vi "Configure - Digital.vi"(5 "master clock channel list":string, 7 "data channel list":string, 8 "error in (no error)":errorcluster, 9 "signal settings":T9, 10 "digital protocol settings":T1={"logic level"=enum."3.3 V", "PCM Data Configuration"={"Frame Sync Edge for Channel 0"=enum."Falling", "Channel Count Per Frame"=2, "Channel Length"=32, "Bit Depth"=24, "Channel 0 Offset"=1, "Endianness"=enum."MSB First", "Data Justification"=enum."Left Justified"}, "bit clock rate"=3025000.0, "master clock rate"=3025000.0, "clock mode"=enum."divided clock", "Frame Sync Clock Control"={"Frame Length"=64, "Frame Sync Pulse Width"=32, "Bit Clock Edge  Sync"=enum."Falling"}} {"master clock rate" format="%.4p"; "bit clock rate" format="%.4p"}, 11 "AudioGeneration in":refnum<class "AudioGeneration.lvclass">) -> (0 "error out":errorcluster, 3 "AudioGeneration out":refnum<class "AudioGeneration.lvclass">)   [LabVIEW 2021, in "AudioGeneration.lvclass"]
uses:
  AudioGeneration.lvclass
  AudioGeneration.lvclass/AudioGeneration.ctl
  <vilib>/NI/STM/TCP/TCP Write Options.ctl
  <vilib>/NI/STM/NI STM.lvlib
  controls/generation type.ctl
  controls/AudioGenTypeDefs.lvlib
  <vilib>/PDM Acquisition Toolkit/host/Classes/Session/Controls/Logic Levels.ctl
  <vilib>/PDM Acquisition Toolkit/host/Classes/Session/DecoderSession.lvclass
  <vilib>/PDM Acquisition Toolkit/shared/controls/Digital Edge.ctl
  <vilib>/PDM Acquisition Toolkit/shared/PDM Shared.lvlib
  <vilib>/PDM Acquisition Toolkit/shared/controls/PCM Bit Endianness.ctl
  <vilib>/PDM Acquisition Toolkit/shared/controls/PCM Data Justification.ctl
  <vilib>/PDM Acquisition Toolkit/shared/controls/PCM Data Format Configuration.ctl
  <vilib>/PDM Acquisition Toolkit/shared/controls/clock mode.ctl
  <vilib>/PDM Acquisition Toolkit/shared/controls/PCM Frame Sync Control.ctl
  controls/digital protocol settings.ctl
  controls/signal type.ctl
  controls/signal settings.ctl
  controls/digital generation settings.ctl
  <vilib>/NI/STM/TCP/Write Message (TCP).vi
  shared/controls/digital output level units.ctl
  shared/controls/audio controls.lvlib
panel:
  out "timeout":bool
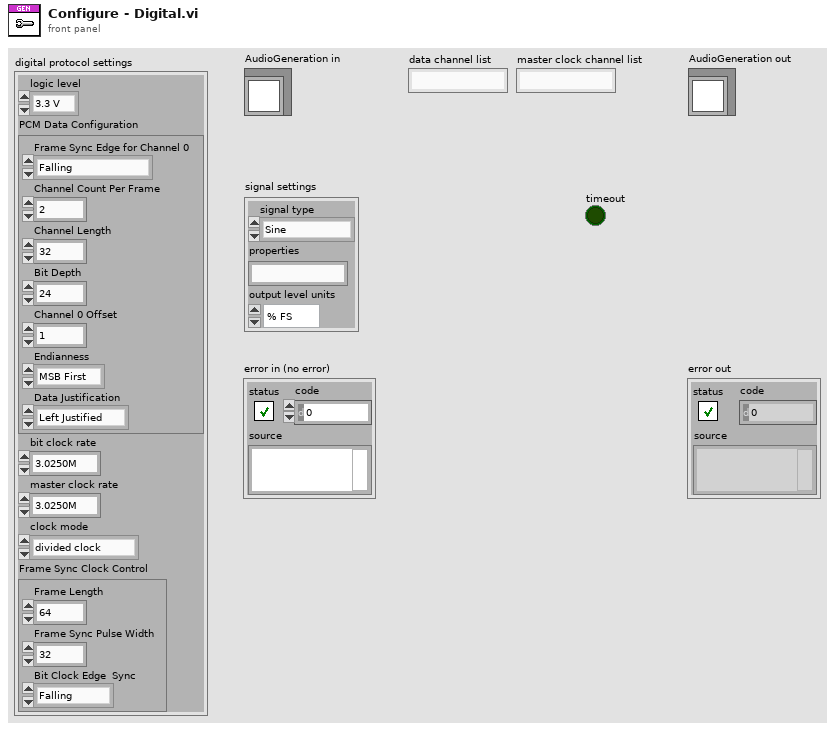
[diagram p1: front panel]
types:
  T1 = typedef "AudioGenTypeDefs.lvlib/digital protocol settings.ctl" = cluster{"logic level":T2, "PCM Data Configuration":T3, "bit clock rate":sgl, "master clock rate":sgl, "clock mode":T7, "Frame Sync Clock Control":T8}
  T2 = typedef "PDM Acquisition Class Library.lvlib/DecoderSession.lvclass/Logic Levels.ctl" = enum16{"3.3 V", "1.8 V", "1.2 V"}
  T3 = typedef "PDM Shared.lvlib/PCM Data Format Configuration.ctl" = cluster{"Frame Sync Edge for Channel 0":T4, "Channel Count Per Frame":u8, "Channel Length":u16, "Bit Depth":u8, "Channel 0 Offset":u16, "Endianness":T5, "Data Justification":T6}
  T4 = typedef "PDM Shared.lvlib/Digital Edge.ctl" = enum8{"Rising", "Falling"}
  T5 = typedef "PDM Shared.lvlib/PCM Bit Endianness.ctl" = enum16{"MSB First", "LSB First"}
  T6 = typedef "PDM Shared.lvlib/PCM Data Justification.ctl" = enum16{"Left Justified", "Right Justified"}
  T7 = typedef "PDM Shared.lvlib/clock mode.ctl" = enum16{"divided clock", "DDS"}
  T8 = typedef "PDM Shared.lvlib/PCM Frame Sync Control.ctl" = cluster{"Frame Length":u16, "Frame Sync Pulse Width":u16, "Bit Clock Edge  Sync":T4}
  T9 = typedef "AudioGenTypeDefs.lvlib/signal settings.ctl" = cluster{"signal type":T10, "properties":string, "output level units":T11}
  T10 = typedef "AudioGenTypeDefs.lvlib/signal type.ctl" = enum16{"Sine", "Dual Tone"}
  T11 = typedef "audio controls.lvlib/digital output level units.ctl" = enum32{"% FS", "dBFS", "V"}
  T12 = typedef "AudioGenTypeDefs.lvlib/digital generation settings.ctl" = cluster{"data channel list":string, "master clock channel list":string, "digital protocol settings":T1, "signal settings":T9}
  T13 = typedef "AudioGenTypeDefs.lvlib/generation type.ctl" = enum16{"analog", "digital"}
  T14 = typedef "NI STM.lvlib/TCP Write Options.ctl" = cluster{"ignore timeout error":bool, "timeout ms (1000)":i32}
  T15 = typedef "NI STM.lvlib/TCP Connection Info.ctl" = cluster{"connection ID":refnum<k5>, "meta data":T16[]}
  T16 = typedef "NI STM.lvlib/MetaDataElement.ctl" = string
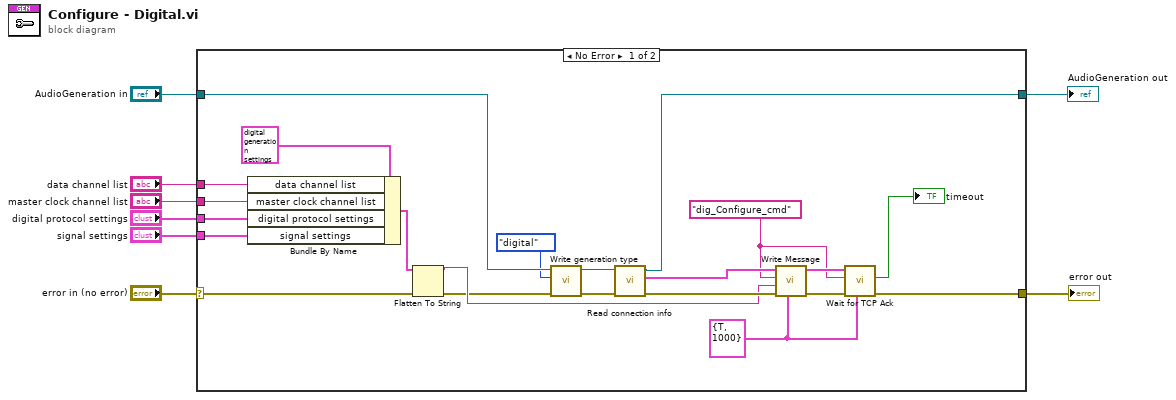
[diagram p0: block diagram]
diagram:
  n1 = case shown="No Error" "error in (no error)" {
    selector: "error in (no error)" -> [w25 w32]
    tunnel: [w27 w32] -> w6
    tunnel: "AudioGeneration in" -> [w20 w31]
    tunnel: [w26 w31] -> w5
    tunnel: "signal settings" -> [w13 _]
    tunnel: "digital protocol settings" -> [w11 _]
    tunnel: "master clock channel list" -> [w10 _]
    tunnel: "data channel list" -> [w9 _]
    frame No Error {
      w16 = "dig_Configure_cmd" ("name")
      w17 = T14 {"ignore timeout error"=TRUE, "timeout ms (1000)"=1000} ("options")
      n2 = Bundle By Name(cluster=T12 {"data channel list"="", "master clock channel list"="", "digital protocol settings"={"logic level"=enum."3.3 V", "PCM Data Configuration"={"Frame Sync Edge for Channel 0"=enum."Falling", "Channel Count Per Frame"=2, "Channel Length"=32, "Bit Depth"=24, "Channel 0 Offset"=1, "Endianness"=enum."MSB First", "Data Justification"=enum."Left Justified"}, "bit clock rate"=3025000.0, "master clock rate"=3025000.0, "clock mode"=enum."divided clock", "Frame Sync Clock Control"={"Frame Length"=64, "Frame Sync Pulse Width"=32, "Bit Clock Edge  Sync"=enum."Falling"}}, "signal settings"={"signal type"=enum."Sine", "properties"="", "output level units"=enum."% FS"}} ("digital generation"), "data channel list"=w9, "master clock channel list"=w10, "digital protocol settings"=w11, "signal settings"=w13) -> (w12:T12)
      n3 = Flatten To String(anything=w12, error in (no error)=w25) -> (data string=w24:string, error out=w23:errorcluster)  [unwired: 2 in, 1 out]
      n4 = call-dynamic "Write generation type.vi"("error in (no error)"=w23, "generation type"=generation_type."digital", "AudioGeneration in"=w20) -> ("error out"=w22:errorcluster, "AudioGeneration out"=w21:refnum<class "AudioGeneration.lvclass">)  [unwired: 7 in]
      n5 = call-dynamic "Read connection info.vi"("error in (no error)"=w22, "AudioGeneration in"=w21) -> ("error out"=w29:errorcluster, "connection info"=w30:T15, "AudioGeneration out"=w26:refnum<class "AudioGeneration.lvclass">)  [unwired: 7 in]
      n6 = call-poly <vilib>:"Write Message.vi"("options"=w17, "error in"=w29, "data"=w24, "name"=w16, "connection info in"=w30) -> ("error out"=w28:errorcluster, "connection info out"=w18:T15)  [unwired: 5 in]
      n7 = call "Wait for TCP Ack.vi"("options"=w17, "error in (no error)"=w28, "cmd name"=w16, "connection info in"=w18) -> ("error out"=w27:errorcluster, "timeout"=→"timeout":bool)  [unwired: 4 in, 2 out]
    }
    frame Error {
    }
  }
  "error out" <- w6
  "AudioGeneration out" <- w5
